vi "Get Generic Slave Module IOVars.vi"(8 "error in (no error)":errorcluster, 11 "ECAT Slave Module in":refnum<k21>="ni.var.io://localhost/EtherCAT Master/Device") -> (0 "error IO":errorcluster, 2 "ECAT Variablenobjekt":refnum<k21>[](array[refnum]))   [LabVIEW 2020, in "SEECD Engine.lvlib"]
uses:
  SEECD Engine.lvlib
  <resource>/objmgr/IndComECAT.rc
  <vilib>/NI VeriStand/Custom Device Tools/Custom Device Utility Library/Custom Device Utility Library.lvlib
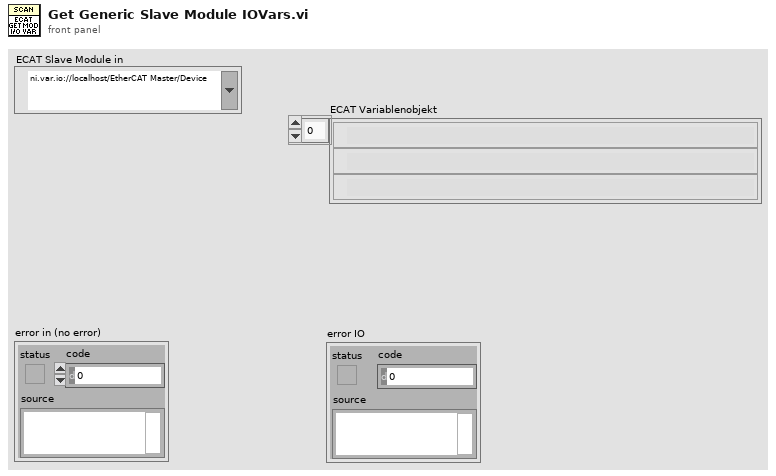
[diagram p1: front panel]
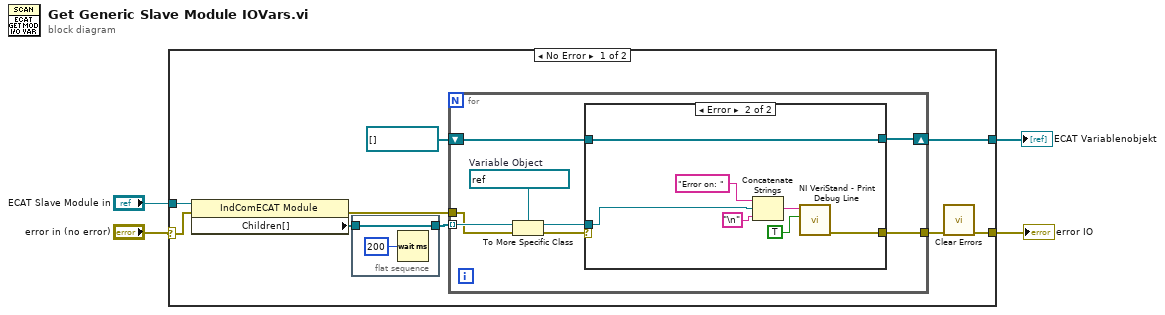
[diagram p0: block diagram]
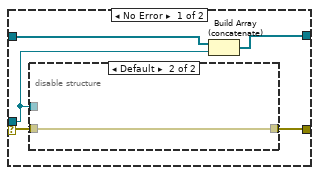
[diagram p2: hidden frame]
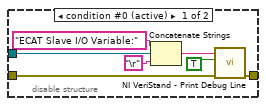
[diagram p3: hidden frame]
diagram:
  n1 = case shown="No Error" "error in (no error)" {
    selector: "error in (no error)" -> [w11 w44]
    tunnel: [w13 w44] -> w1
    tunnel: "ECAT Slave Module in" -> [w12 _]
    tunnel: [w5 _] -> w2
    frame No Error {
      n2 = property class="IndComECAT Module"(reference=w12, error in=w11) -> (error out=w10:errorcluster, "Children[]"=w8:refnum<k21>[])  [unwired: 1 out]
      n3 = flat-sequence {
        tunnel: w8 -> [w15]
        tunnel: [w15] -> w7
        frame #0 {
          n4 = Wait (ms)(milliseconds to wait=u32 200) -> ()  [unwired: 1 out]
        }
      }
      n5 = for {
        tunnel: w7 -> [w20] mode=indexing
        tunnel: w10 -> [w16]
        tunnel: [w23] -> w9
        shift-right: [w22] -> w5
        shift-left: refnum<k21>[] [] -> [w21]
        w17 = refnum<k21> refnum  # Variable Object
        n6 = To More Specific Class(target class=w17, reference=w20, error in=w16) -> (specific class reference=w18:refnum<k21>, error out=w19:errorcluster)
        n7 = case shown="Error" w19 {
          selector: w19 -> [w24 _]
          tunnel: w18 -> [w26 w38]
          tunnel: [w25 w40] -> w23
          tunnel: [w27 w43] -> w22
          tunnel: w21 -> [w28 w43]
          frame No Error {
            n8 = disable-structure shown="Default" {
              disable-tunnel: w26 -> [w35 _]
              disable-tunnel: [w33 w36] -> w25
              disable-tunnel: w24 -> [w32 w36]
              frame condition #0 (active) {
                n9 = Concatenate Strings("ECAT Slave I/O Variable:", w35, "\r") -> (w31:string)
                n10 = call <vilib>:"NI VeriStand - Print Debug Line.vi"("error in (no error)"=w32, "Add to log file? (F)"=TRUE, "Message"=w31) -> ("error out"=w33:errorcluster)  [unwired: 8 in]
              }
              frame condition #1 {
              }
            }
            n11 = Build Array (concatenate)(w28, w26) -> (w27:refnum<k21>[])
          }
          frame Error {
            n12 = Concatenate Strings("Error on: ", w38, "\n") -> (w41:string)
            n13 = call <vilib>:"NI VeriStand - Print Debug Line.vi"("Add to log file? (F)"=TRUE ("Add to log file? (T)"), "Message"=w41) -> ("error out"=w40:errorcluster)  [unwired: 9 in]
          }
        }
      }
      n14 = call <vilib>:"Clear Errors.vi"("error in (no error)"=w9) -> ("error out"=w13:errorcluster)  [unwired: 5 in, 1 out]
    }
    frame Error {
    }
  }
  "error IO" <- w1
  "ECAT Variablenobjekt" <- w2
